vi "Template Change Field IDs for INI Export.vi"(8 "error in (no error)":errorcluster, 10 "Parameters":T2, 11 "Connection Refnum":T1) -> (0 "error out":errorcluster, 2 "Parameters 2":T2, 3 "Connection Refnum 2":T1)   [LabVIEW 2011]
uses:
  Addons/internet/utils/keyedarr.llb/Keyed Array.ctl
  SI.LIB/ODBC/SQL Controls/Connection Refnum.ctl
  Addons/internet/utils/strutil.llb/Case Matching.ctl
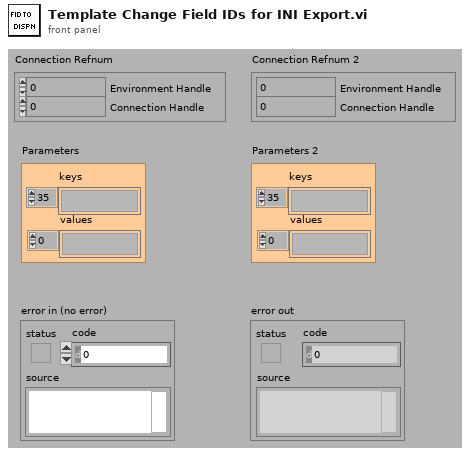
[diagram p1: front panel]
types:
  T1 = typedef "Connection Refnum.ctl" = cluster{"Environment Handle":i32, "Connection Handle":i32}
  T2 = typedef "Keyed Array.ctl" = cluster{"keys":string[], "values":string[]}
  T3 = typedef "Case Matching.ctl" = enum16{"a != A", "a == A", "system"}
  T4 = typedef "Field Record.ctl" = cluster{"ixField":i32, "iSequenceOrder":i32, "sxFieldId":string, "sxSequenceId":string, "sDisplayName":string, "sValue":string, "sUnits":string, "nDataType":T5, "nNextItem":T6, "fSystem":bool, "fSystemValue":bool, "fRequired":bool, "fSetAtTest":bool, "fTestField":bool, "fDeleted":bool, "fIndexed":bool, "fFreeList":bool}
  T5 = typedef "Field DataTypes.ctl" = enum32{"text", "numeric", "list", "timestamp", "boolean"}
  T6 = typedef "Field NextItem.ctl" = enum32{"Reset", "Retain", "Auto-Increment"}
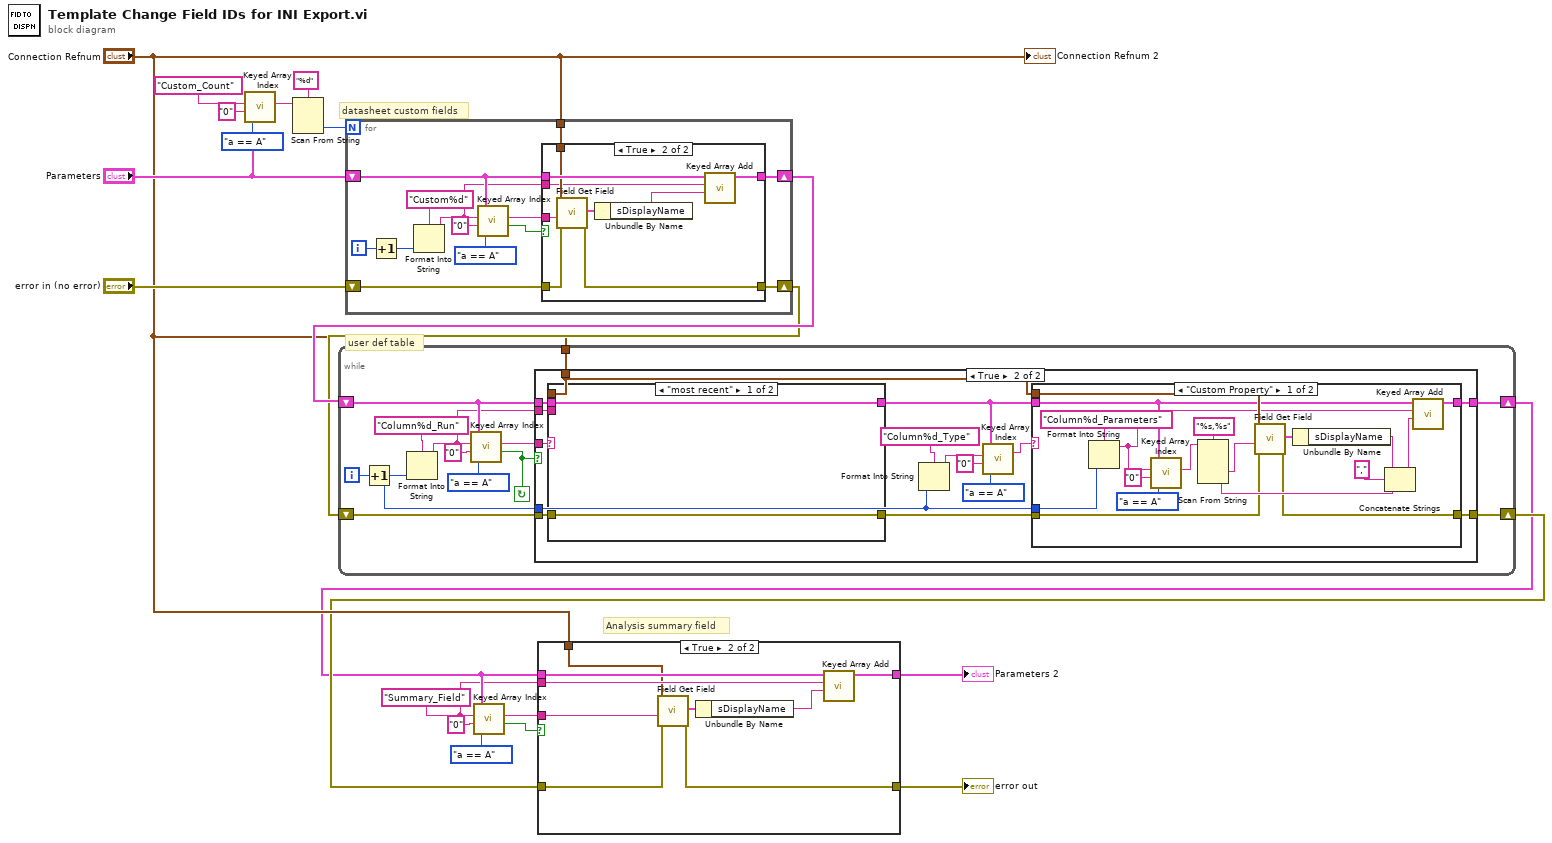
[diagram p0: block diagram]
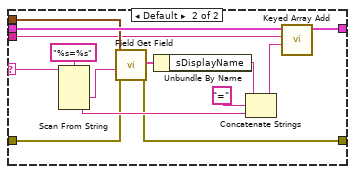
[diagram p5: hidden frame]
diagram:
  w1 = "Summary_Field" ("key")
  # "Analysis summary field"
  # "user def table"
  # "datasheet custom fields"
  n1 = call "Keyed Array Index.vi"("case matching (sensitive)"=Case_Matching."a == A", "default value"="0", "key"="Custom_Count", "array in"="Parameters") -> ("value"=w16:string)  [unwired: 3 out]
  n2 = Scan From String(format string="%d", input string=w16) -> (output 1=w17:i32)  [unwired: 2 in, 4 out]
  n3 = for {
    N: w17 -> [_]
    tunnel: "Connection Refnum" -> [w27]
    shift-right: [w24] -> w11
    shift-left: "error in (no error)" -> [w25]
    shift-right: [w21] -> w12
    shift-left: "Parameters" -> [w28]
    i -> [w30]
    n4 = Increment(x=w30) -> (x+1=w29:i32)
    n5 = Format Into String(format string="Custom%d" ("key"), w29) -> (resulting string=w23:string)  [unwired: 2 in, 1 out]
    n6 = call "Keyed Array Index.vi"("case matching (sensitive)"=Case_Matching."a == A", "default value"="0", "key"=w23, "array in"=w28) -> ("valid key"=w22:bool, "value"=w26:string)  [unwired: 2 out]
    n7 = case shown="True" w22 {
      tunnel: w28 -> [w34 w44]
      tunnel: w27 -> [_ w43]
      tunnel: w26 -> [_ w42]
      tunnel: w25 -> [w35 w41]
      tunnel: [w35 w40] -> w24
      tunnel: w23 -> [_ w38]
      tunnel: [w34 w36] -> w21
      frame False {
      }
      frame True {
        n8 = call "Field Get Field.vi"("error in (no error)"=w41, "sFieldId or sDisplayName (\"\")"=w42, "Connection Refnum"=w43) -> ("error out"=w40:errorcluster, "Field"=w39:T4)  [unwired: 2 in, 5 out]
        n9 = Unbundle By Name(w39) -> ("sDisplayName"=w37:string)
        n10 = call "Keyed Array Add.vi"("value"=w37, "key"=w38, "array in"=w44) -> ("array out"=w36:T2)  [unwired: 1 in, 3 out]
      }
    }
  }
  n11 = while {
    tunnel: "Connection Refnum" -> [w52]
    shift-right: [w45] -> w9
    shift-left: w11 -> [w50]
    shift-right: [w48] -> w8
    shift-left: w12 -> [w53]
    i -> [w54]
    stop <- w47 continue-if-true
    n12 = Increment(x=w54) -> (x+1=w46:i32)
    n13 = Format Into String(format string="Column%d_Run" ("key"), w46) -> (resulting string=w49:string)  [unwired: 2 in, 1 out]
    n14 = call "Keyed Array Index.vi"("case matching (sensitive)"=Case_Matching."a == A", "default value"="0", "key"=w49, "array in"=w53) -> ("valid key"=w47:bool, "value"=w51:string)  [unwired: 2 out]
    n15 = case shown="True" w47 {
      tunnel: w53 -> [w59 w74]
      tunnel: w52 -> [_ w63]
      tunnel: w51 -> [_ w72]
      tunnel: w50 -> [w58 w68]
      tunnel: w49 -> [_ w73]
      tunnel: [w59 w65] -> w48
      tunnel: w46 -> [_ w61]
      tunnel: [w58 w64] -> w45
      frame False {
      }
      frame True {
        n16 = case shown="\"most recent\"" w72 {
          selector: w72 -> [_ w105]
          tunnel: w74 -> [w96 w110]
          tunnel: w63 -> [_ w109]
          tunnel: w73 -> [_ w107]
          tunnel: [w96 w106] -> w66
          tunnel: w68 -> [w95 w98]
          tunnel: [w95 w97] -> w67
          frame "most recent" {
          }
          frame Default {
            n17 = Scan From String(format string="%s=%s", input string=w105) -> (output 1=w103:string, output 2=w100:string)  [unwired: 2 in, 5 out]
            n18 = call "Field Get Field.vi"("error in (no error)"=w98, "sFieldId or sDisplayName (\"\")"=w103, "Connection Refnum"=w109) -> ("error out"=w97:errorcluster, "Field"=w108:T4)  [unwired: 2 in, 5 out]
            n19 = Unbundle By Name(w108) -> ("sDisplayName"=w102:string)
            n20 = Concatenate Strings(w102, "=" ("format string"), w100) -> (w101:string)
            n21 = call "Keyed Array Add.vi"("value"=w101, "key"=w107, "array in"=w110) -> ("array out"=w106:T2)  [unwired: 1 in, 3 out]
          }
        }
        n22 = Format Into String(format string="Column%d_Type" ("key"), w61) -> (resulting string=w71:string)  [unwired: 2 in, 1 out]
        n23 = call "Keyed Array Index.vi"("case matching (sensitive)"=Case_Matching."a == A", "default value"="0", "key"=w71, "array in"=w66) -> ("value"=w62:string)  [unwired: 3 out]
        n24 = case shown="\"Custom Property\"" w62 {
          tunnel: w66 -> [w78 w94]
          tunnel: w63 -> [w92 _]
          tunnel: [w90 w94] -> w65
          tunnel: w67 -> [w83 w93]
          tunnel: [w82 w93] -> w64
          tunnel: w61 -> [w80 _]
          frame "Custom Property" {
            n25 = Format Into String(format string="Column%d_Parameters" ("key"), w80) -> (resulting string=w75:string)  [unwired: 2 in, 1 out]
            n26 = call "Keyed Array Index.vi"("case matching (sensitive)"=Case_Matching."a == A", "default value"="0", "key"=w75, "array in"=w78) -> ("value"=w77:string)  [unwired: 3 out]
            n27 = Scan From String(format string="%s,%s", input string=w77) -> (output 1=w88:string, output 2=w85:string)  [unwired: 2 in, 5 out]
            n28 = call "Field Get Field.vi"("error in (no error)"=w83, "sFieldId or sDisplayName (\"\")"=w88, "Connection Refnum"=w92) -> ("error out"=w82:errorcluster, "Field"=w91:T4)  [unwired: 2 in, 5 out]
            n29 = Unbundle By Name(w91) -> ("sDisplayName"=w87:string)
            n30 = Concatenate Strings(w87, "," ("format string"), w85) -> (w86:string)
            n31 = call "Keyed Array Add.vi"("value"=w86, "key"=w75, "array in"=w78) -> ("array out"=w90:T2)  [unwired: 1 in, 3 out]
          }
          frame Default {
          }
        }
      }
    }
  }
  n32 = call "Keyed Array Index.vi"("case matching (sensitive)"=Case_Matching."a == A", "default value"="0", "key"=w1, "array in"=w8) -> ("valid key"=w4:bool, "value"=w5:string)  [unwired: 2 out]
  n33 = case shown="True" w4 {
    tunnel: w8 -> [w112 w121]
    tunnel: "Connection Refnum" -> [_ w118]
    tunnel: w5 -> [_ w116]
    tunnel: w9 -> [w111 w119]
    tunnel: w1 -> [_ w120]
    tunnel: [w112 w113] -> w3
    tunnel: [w111 w114] -> w2
    frame False {
    }
    frame True {
      n34 = call "Field Get Field.vi"("error in (no error)"=w119, "sFieldId or sDisplayName (\"\")"=w116, "Connection Refnum"=w118) -> ("error out"=w114:errorcluster, "Field"=w117:T4)  [unwired: 2 in, 5 out]
      n35 = Unbundle By Name(w117) -> ("sDisplayName"=w115:string)
      n36 = call "Keyed Array Add.vi"("value"=w115, "key"=w120, "array in"=w121) -> ("array out"=w113:T2)  [unwired: 1 in, 3 out]
    }
  }
  "Parameters 2" <- w3
  "error out" <- w2
  "Connection Refnum 2" <- "Connection Refnum"
